vi "Update_Results.vi"(8 "error in (no error)":errorcluster, 9 "Results Array In":dbl[](array[numeric]), 10 "ControlWord In":u16 format="%08b", 11 "SoftmotionAxis in":refnum<class "SoftmotionAxis.lvclass">) -> (0 "error out":errorcluster, 1 "appended array":dbl[](array[numeric]), 3 "SoftmotionAxis out":refnum<class "SoftmotionAxis.lvclass">)   [LabVIEW 2017, in "SoftmotionAxis.lvclass"]
uses:
  SoftmotionAxis.lvclass
  Utilities/Bit Manipulation.lvlib
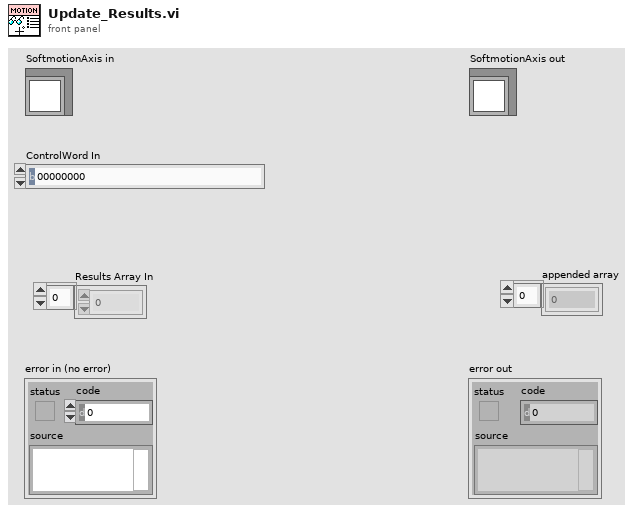
[diagram p1: front panel]
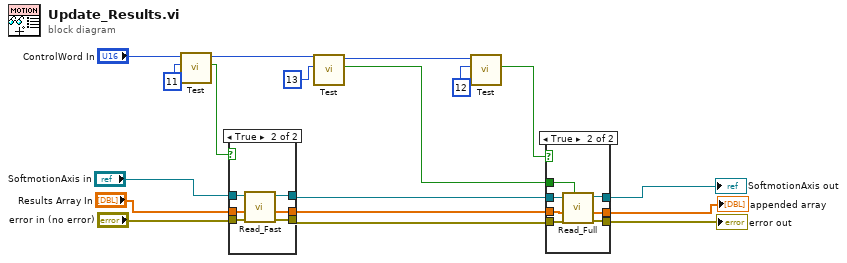
[diagram p0: block diagram]
diagram:
  n1 = call "Test.vi"("Bit to test"=u8 11, "Data_In"="ControlWord In") -> ("bit value"=w18:bool, "Data_Out"=w3:u16)  [unwired: 8 in]
  n2 = case shown="True" w18 {
    tunnel: [w19 w22] -> w12
    tunnel: [w20 w27] -> w13
    tunnel: [w21 w26] -> w14
    tunnel: "SoftmotionAxis in" -> [w21 w25]
    tunnel: "error in (no error)" -> [w20 w24]
    tunnel: "Results Array In" -> [w19 w23]
    frame False {
    }
    frame True {
      n3 = call-dynamic "Read_Fast.vi"("error in (no error)"=w24, "Results Array In"=w23, "SoftmotionAxis in"=w25) -> ("error out"=w27:errorcluster, "appended array"=w22:dbl[], "SoftmotionAxis out"=w26:refnum<class "SoftmotionAxis.lvclass">)  [unwired: 6 in]
    }
  }
  n4 = call "Test.vi"("Bit to test"=u8 13, "Data_In"=w3) -> ("bit value"=w5:bool, "Data_Out"=w2:u16)  [unwired: 8 in]
  n5 = call "Test.vi"("Bit to test"=u8 12, "Data_In"=w2) -> ("bit value"=w15:bool)  [unwired: 8 in, 1 out]
  n6 = case shown="True" w15 {
    tunnel: [w29 w34] -> w7
    tunnel: [w30 w36] -> w8
    tunnel: w14 -> [w30 w37]
    tunnel: w13 -> [w29 w35]
    tunnel: w12 -> [w28 w33]
    tunnel: [w28 w32] -> w6
    tunnel: w5 -> [_ w31]
    frame False {
    }
    frame True {
      n7 = call-dynamic "Read_Full.vi"("CheckFaults"=w31, "error in (no error)"=w35, "Results Array In"=w33, "SoftmotionAxis in"=w37) -> ("error out"=w34:errorcluster, "appended array"=w32:dbl[], "SoftmotionAxis out"=w36:refnum<class "SoftmotionAxis.lvclass">)  [unwired: 5 in]
    }
  }
  "error out" <- w7
  "SoftmotionAxis out" <- w8
  "appended array" <- w6
